vi "Limit Position Write.vi"(4 "error in (no error)":errorcluster, 5 "Value":cluster{"Lower Limit":dbl, "Upper Limit":dbl}, 6 "Container State":T2, 7 "Display State In":T1={"Numeric"=0.0, "Fill Plots"=FALSE, "Cursor Redraw"=TRUE, "XYGraph Refnum"=refnum}) -> (0 "error out":errorcluster, 3 "Display State Out":T1={"Numeric"=0.0, "Fill Plots"=FALSE, "Cursor Redraw"=TRUE, "XYGraph Refnum"=refnum})   [LabVIEW 2020, in "Overview XControl.xctl"]
uses:
  Overview XControl.xctl
  <vilib>/_xctls/Container State.ctl
  Overview State.ctl
  <vilib>/_xctls/XControlSupport.lvlib
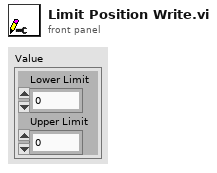
[diagram p1: front panel]
types:
  T1 = typedef "Overview XControl.xctl/Overview State.ctl" = cluster{"Numeric":dbl, "Fill Plots":bool, "Cursor Redraw":bool, "XYGraph Refnum":refnum<vi>}
  T2 = typedef "XControlSupport.lvlib/Container State.ctl" = cluster{"Indicator?":bool, "Run Mode?":bool, " Refnum":refnum<vi>}
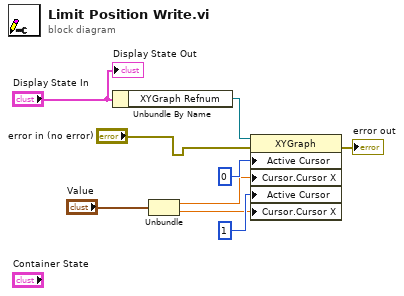
[diagram p0: block diagram]
diagram:
  n1 = Unbundle By Name("Display State In") -> ("XYGraph Refnum"=w6:refnum<vi>)
  n2 = Unbundle("Value") -> ("Lower Limit"=w3:dbl, "Upper Limit"=w2:dbl)
  n3 = property class="XYGraph"(reference=w6, error in="error in (no error)", "Active Cursor"=u32 0, "Cursor.Cursor X"=w3, "Active Cursor"=u32 1, "Cursor.Cursor X"=w2) -> (error out=→"error out":errorcluster)  [unwired: 1 out]
  "Display State Out" <- "Display State In"
